vi "svc_Sort XY Results.vi"(9 "sort order":u16(ring) items=["Ascending", "Descending"], 10 "sort by":u16(ring) items=["X", "Y"], 11 "XY in":cluster{"X":dbl[], "Y":dbl[]}) -> (2 "sort indices":i32[](array[numeric]), 3 "sorted XY":cluster{"X":dbl[], "Y":dbl[]})   [LabVIEW 2017]
doc: "Sorts an array of peaks according to the <B>sort by</B> and <B>sort order</B> parameters. Use this VI to sort peaks that the SVFA Spectrum Peak Search, SVT Spurious Free Dynamic Range, and SVT THD and Harmonic Components VIs return. Wire data to the<B> peaks in</B> input to determine the polymorphic instance to use or manually select the instance."
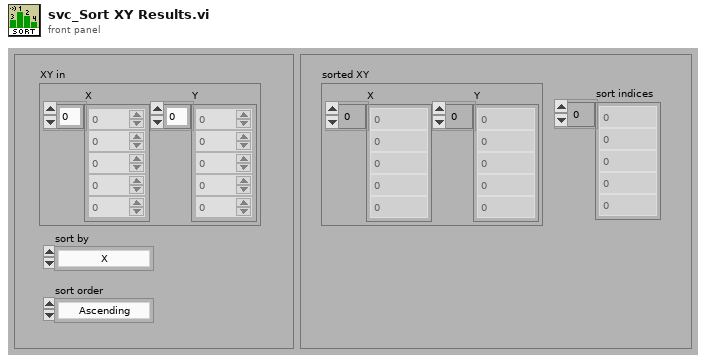
[diagram p1: front panel]
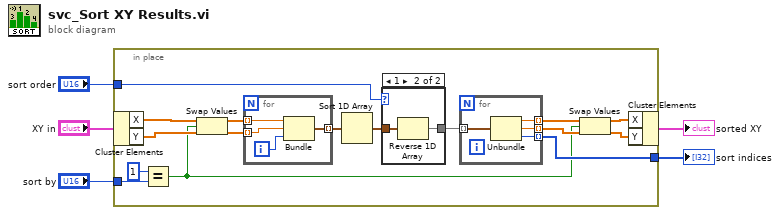
[diagram p0: block diagram]
diagram:
  n1 = in-place {
    in-place-border: "sort order" -> [w20]
    in-place-border: [w17] -> w4
    in-place-border: "sort by" -> [w16]
    n2 = in-place-cluster #1("XY in") -> ("X"=w14:dbl[], "Y"=w13:dbl[])
    n3 = Equal?(x=u16 1 ("y"), y=w16) -> (x = y?=w7:bool)
    n4 = Swap Values(12:w14, 13:w7, 14:w13) -> (1:w12:dbl[], 3:w11:dbl[])
    n5 = for {
      tunnel: w12 -> [w25] mode=indexing
      tunnel: w11 -> [w24] mode=indexing
      tunnel: [w23] -> w19 mode=indexing
      i -> [w22]
      n6 = Bundle(w25, w24, w22) -> (w23:cluster{dbl, dbl, i32})  [unwired: 1 in]
    }
    n7 = Sort 1D Array(array=w19) -> (sorted array=w21:cluster{dbl, dbl, i32}[])
    n8 = case shown="1" w20 {
      tunnel: [w30 w31] -> w18
      tunnel: w21 -> [w30 w32]
      frame 0, Default {
      }
      frame 1 {
        n9 = Reverse 1D Array(array=w32) -> (reversed array=w31:cluster{dbl, dbl, i32}[])
      }
    }
    n10 = for {
      tunnel: w18 -> [w29] mode=indexing
      tunnel: [w28] -> w10 mode=indexing
      tunnel: [w27] -> w8 mode=indexing
      tunnel: [w26] -> w17 mode=indexing
      n11 = Unbundle(w29) -> (w28:dbl, w27:dbl, w26:i32)
    }
    n12 = Swap Values(12:w10, 13:w7, 14:w8) -> (1:w9:dbl[], 3:w6:dbl[])
    n13 = in-place-cluster #1("X"=w9, "Y"=w6) -> (→"sorted XY":cluster{"X":dbl[], "Y":dbl[]})
  }
  "sort indices" <- w4
